vi "Steps2deg_power.vi"(8 "Max_power":dbl, 9 "Min_power":dbl, 10 "Min_angle":dbl, 11 "Steps":i32) -> (2 "Power":dbl, 3 "Deg":dbl)   [LabVIEW 2012]
panel:
  in  "Offset":i32
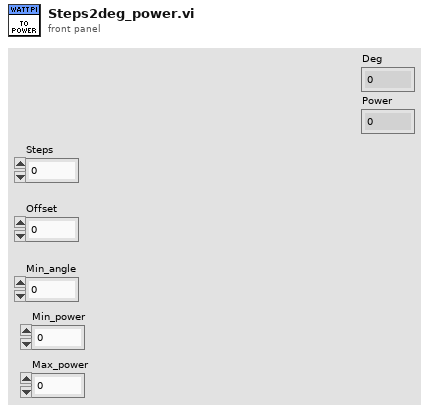
[diagram p1: front panel]
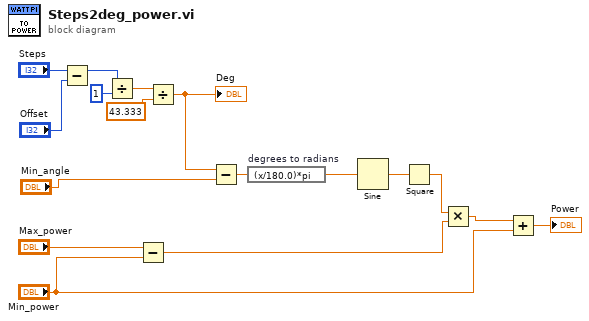
[diagram p0: block diagram]
diagram:
  n1 = Subtract(x="Steps", y="Offset") -> (x-y=w13:i32)
  n2 = Divide(x=w13, y=1) -> (x/y=w15:dbl)
  n3 = Subtract(x="Max_power", y="Min_power") -> (x-y=w4:dbl)
  n4 = Divide(x=w15, y=43.333) -> (x/y=w11:dbl)
  "Deg" <- w11
  n5 = Subtract(x=w11, y="Min_angle") -> (x-y=w9:dbl)
  n6 = expression code="(x/180.0)*pi" "degrees to radians"(w9) -> (w8:dbl)
  n7 = Sine(x=w8) -> (sin(x)=w7:dbl)
  n8 = Square(x=w7) -> (x^2=w5:dbl)
  n9 = Multiply(x=w5, y=w4) -> (x*y=w3:dbl)
  n10 = Add(x=w3, y="Min_power") -> (x+y=→"Power":dbl)
